vi "Configure Controlled TimerDRV.vi"(5 "Processor Core":i32=-2, 7 "Target Frequency":dbl=100.0, 8 "error in (no error)":errorcluster, 10 "Target Type":T1=enum."Windows", 11 "TimerDRV in":refnum<class "TimerDRV.lvclass">) -> (0 "error out":errorcluster, 3 "TimerDRV out":refnum<class "TimerDRV.lvclass">)   [LabVIEW 2019, in "TimingDRV Engine.lvlib" / "TimerDRV.lvclass"]
uses:
  TimerDRV.lvclass
  TypeDefs/Target Type.ctl
  TimerDRV.lvclass/TimerDRV.ctl
  <vilib>/Utility/error.llb/Error Cluster From Error Code.vi
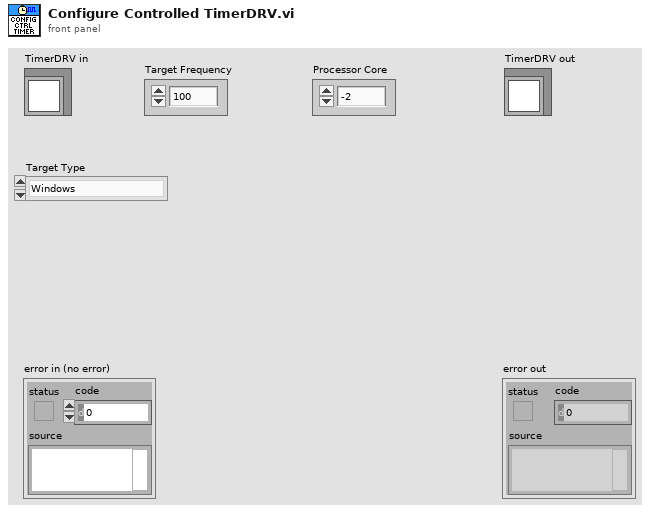
[diagram p1: front panel]
types:
  T1 = typedef "TimingDRV Engine.lvlib/TimerDRV.lvclass/Target Type.ctl" = enum16{"PharLap", "VxWorks", "Windows", "Linux_32_ARM", "Linux_x64"}
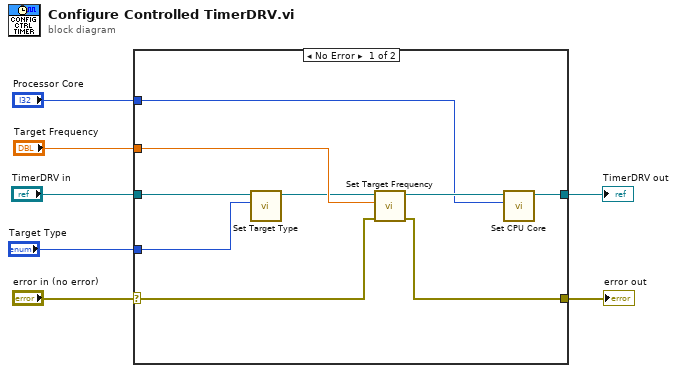
[diagram p0: block diagram]
diagram:
  n1 = case shown="No Error" "error in (no error)" {
    selector: "error in (no error)" -> [w9 w18]
    tunnel: [w8 w18] -> w6
    tunnel: [w13 w17] -> w4
    tunnel: "TimerDRV in" -> [w12 w17]
    tunnel: "Target Frequency" -> [w16 _]
    tunnel: "Processor Core" -> [w14 _]
    tunnel: "Target Type" -> [w10 _]
    frame No Error {
      n2 = call "Set Target Type.vi"("Target Type"=w10, "TimerDRV in"=w12) -> ("TimerDRV out"=w11:refnum<class "TimerDRV.lvclass">)  [unwired: 9 in]
      n3 = call "Set Target Frequency.vi"("Error In"=w9, "Target Frequency"=w16, "TimerDRV in"=w11) -> ("Error Out"=w8:errorcluster, "TimerDRV out"=w15:refnum<class "TimerDRV.lvclass">)  [unwired: 7 in]
      n4 = call "Set CPU Core.vi"("CPU Core"=w14, "TimerDRV in"=w15) -> ("TimerDRV out"=w13:refnum<class "TimerDRV.lvclass">)  [unwired: 9 in]
    }
    frame Error {
    }
  }
  "error out" <- w6
  "TimerDRV out" <- w4
